vi "Decrease goods subvi.vi"(10 "Status":T2, 11 "Order":T1) -> (3 "Cluster":T2)   [LabVIEW 2020]
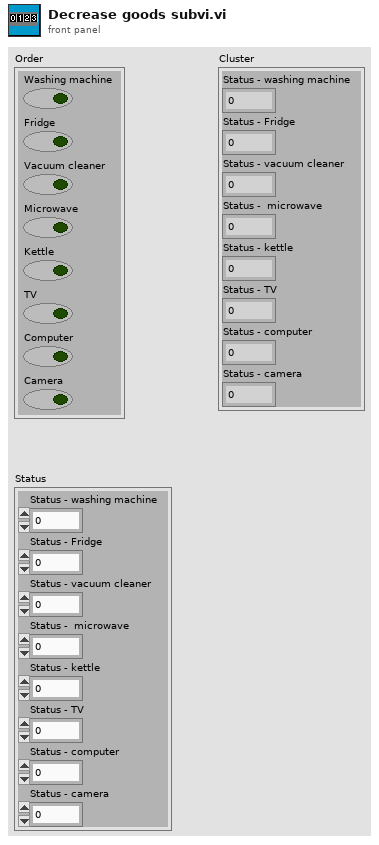
[diagram p1: front panel]
types:
  T1 = cluster{"Washing machine":bool, "Fridge":bool, "Vacuum cleaner":bool, "Microwave":bool, "Kettle":bool, "TV":bool, "Computer":bool, "Camera":bool}
  T2 = cluster{"Status - washing machine":u32, "Status - Fridge":u32, "Status - vacuum cleaner":u32, "Status -  microwave":u32, "Status - kettle":u32, "Status - TV":u32, "Status - computer":u32, "Status - camera":u32}
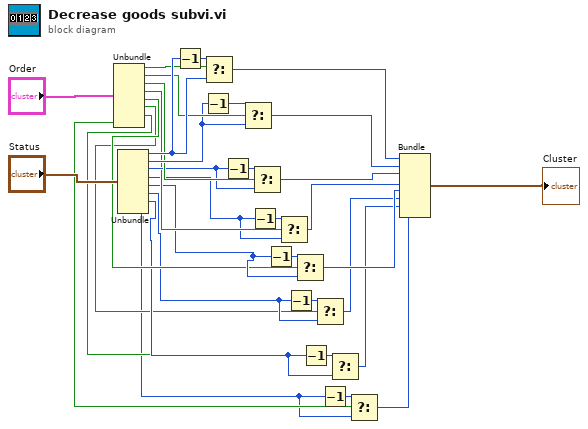
[diagram p0: block diagram]
diagram:
  n1 = Unbundle("Order") -> ("Washing machine"=w31:bool, "Fridge"=w26:bool, "Vacuum cleaner"=w22:bool, "Microwave"=w18:bool, "Kettle"=w13:bool, "Computer"=w6:bool, "Camera"=w3:bool)  [unwired: 1 out]
  n2 = Unbundle("Status") -> ("Status - washing machine"=w34:u32, "Status - Fridge"=w25:u32, "Status - vacuum cleaner"=w21:u32, "Status -  microwave"=w17:u32, "Status - kettle"=w14:u32, "Status - TV"=w10:u32, "Status - computer"=w7:u32, "Status - camera"=w2:u32)
  n3 = Decrement(x=w34) -> (x-1=w33:u32)
  n4 = Decrement(x=w25) -> (x-1=w27:u32)
  n5 = Select(t=w33, s=w31, f=w34) -> (s? t:f=w32:u32)
  n6 = Decrement(x=w21) -> (x-1=w23:u32)
  n7 = Select(t=w27, s=w26, f=w25) -> (s? t:f=w24:u32)
  n8 = Decrement(x=w17) -> (x-1=w19:u32)
  n9 = Select(t=w23, s=w22, f=w21) -> (s? t:f=w20:u32)
  n10 = Decrement(x=w14) -> (x-1=w15:u32)
  n11 = Select(t=w19, s=w18, f=w17) -> (s? t:f=w16:u32)
  n12 = Decrement(x=w10) -> (x-1=w11:u32)
  n13 = Select(t=w15, s=w13, f=w14) -> (s? t:f=w12:u32)
  n14 = Decrement(x=w7) -> (x-1=w8:u32)
  n15 = Select(t=w11, s=w6, f=w10) -> (s? t:f=w9:u32)
  n16 = Decrement(x=w2) -> (x-1=w4:u32)
  n17 = Select(t=w8, s=w6, f=w7) -> (s? t:f=w5:u32)
  n18 = Select(t=w4, s=w3, f=w2) -> (s? t:f=w1:u32)
  n19 = Bundle("Status - washing machine"=w32, "Status - Fridge"=w24, "Status - vacuum cleaner"=w20, "Status -  microwave"=w16, "Status - kettle"=w12, "Status - TV"=w9, "Status - computer"=w5, "Status - camera"=w1) -> (→"Cluster":T2)  [unwired: 1 in]
